vi "Read Control Box.vi"(6 "Timeout?":bool, 8 "error in (no error)":errorcluster, 9 "Bad Packet?":bool, 10 "Raw Data":u8[](array[numeric]) format="%.0x", 11 "Control Box in":refnum<class "Control Box.lvclass">) -> (0 "error out":errorcluster, 1 "Remaining Channels":T1[](array[typedef]), 2 "Control Board":T1, 3 "Control Box out":refnum<class "Control Box.lvclass">)   [LabVIEW 2018, in "Control Box.lvlib" / "Control Box.lvclass"]
uses:
  Control Box.lvclass
  Custom Controls/Channel Status.ctl
  Control Box.lvclass/Control Box.ctl
  Control Box.lvlib
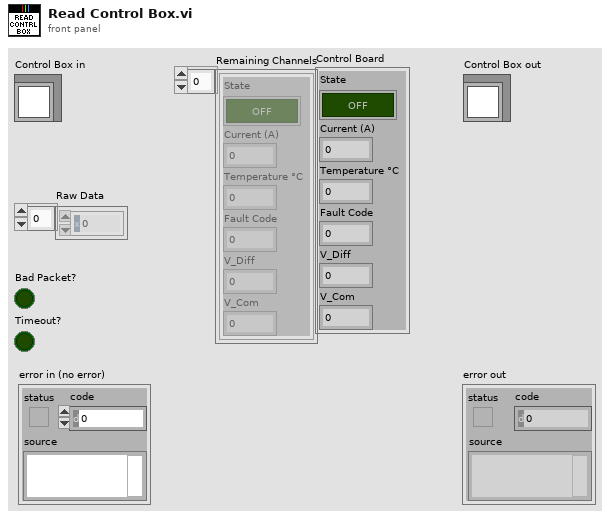
[diagram p1: front panel]
types:
  T1 = typedef "Control Box.lvlib/Channel Status.ctl" = cluster{"State":bool, "Current (A)":dbl, "Temperature °C":dbl, "Fault Code":u8, "V_Diff":dbl, "V_Com":dbl}
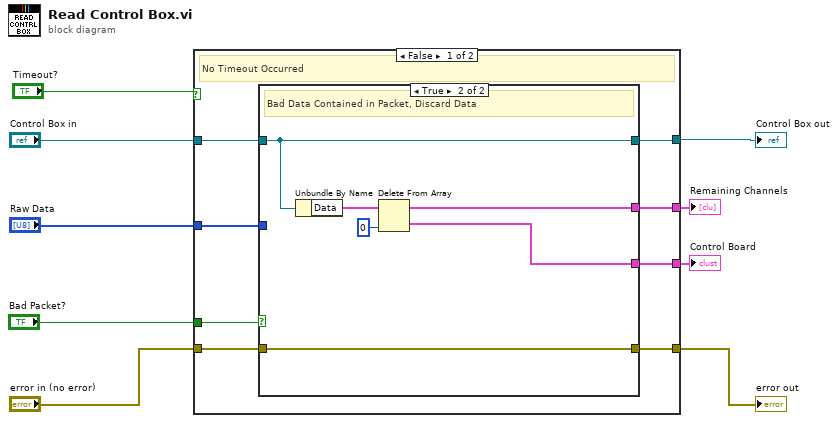
[diagram p0: block diagram]
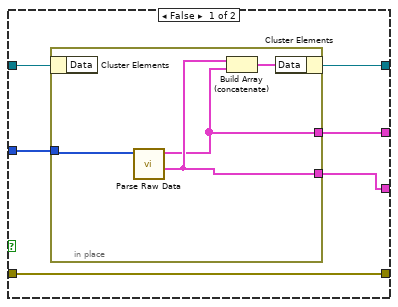
[diagram p2: hidden frame]
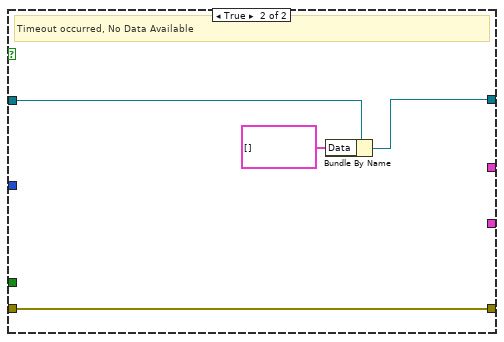
[diagram p3: hidden frame]
diagram:
  n1 = case shown="False" "Timeout?" {
    tunnel: "Control Box in" -> [w14 w37]
    tunnel: [w13 w36] -> w7
    tunnel: "error in (no error)" -> [w17 w34]
    tunnel: [w15 w34] -> w5
    tunnel: "Bad Packet?" -> [w16 _]
    tunnel: [w12 _] -> w3
    tunnel: [w11 _] -> w2
    tunnel: "Raw Data" -> [w10 _]
    frame False {
      # "No Timeout Occurred"
      n2 = case shown="True" w16 {
        tunnel: w17 -> [w18 w33]
        tunnel: [w18 w33] -> w15
        tunnel: w14 -> [w23 w32]
        tunnel: [w21 w32] -> w13
        tunnel: [w19 w29] -> w12
        tunnel: [w20 w28] -> w11
        tunnel: w10 -> [w22 _]
        frame False {
          n3 = in-place {
            in-place-border: w22 -> [w27]
            in-place-border: [w24] -> w20
            in-place-border: [w25] -> w19
            n4 = in-place-cluster #1(w23) -> ()  [unwired: 1 out]
            n5 = call "Parse Raw Data.vi"("Raw Data"=w27) -> ("Board Out"=w25:T1, "Modules Out"=w24:T1[])  [unwired: 9 in]
            n6 = Build Array (concatenate)(w25, w24) -> (w26:T1[])
            n7 = in-place-cluster #1("Data"=w26) -> (w21:refnum<class "Control Box.lvclass">)
          }
        }
        frame True {
          # "Bad Data Contained in Packet, Discard Data"
          n8 = Unbundle By Name(w32) -> ("Data"=w31:T1[])
          n9 = Delete From Array(array=w31, index=0) -> (deleted portion=w29:T1, array with subset deleted=w28:T1[])  [unwired: 1 in]
        }
      }
    }
    frame True {
      # "Timeout occurred, No Data Available"
      n10 = Bundle By Name(cluster=w37, "Data"=T1[] []) -> (w36:refnum<class "Control Box.lvclass">)
    }
  }
  "error out" <- w5
  "Control Box out" <- w7
  "Control Board" <- w3
  "Remaining Channels" <- w2
